vi "Helper - detect wind cross.vi"(10 "Heading Change":dbl, 11 "Apparent Wind":T1) -> (3 "Crossing Wind?":bool)   [LabVIEW 2011]
doc: "Checks whether the boat wants to cross the wind. Takes in the difference between optimal heading and current heading and the apparent wind. Returns true if the boat wants to cross the wind."
uses:
  2 Typedefs/apparent wind.ctl
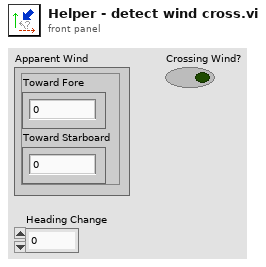
[diagram p1: front panel]
types:
  T1 = typedef "apparent wind.ctl" = cluster{"Toward Fore":dbl, "Toward Starboard":dbl}
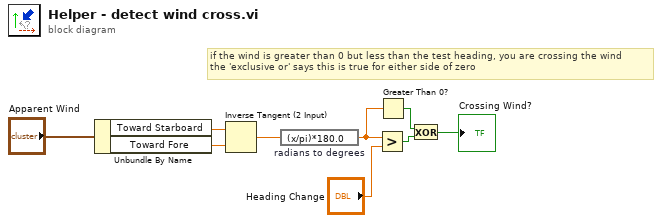
[diagram p0: block diagram]
diagram:
  # "if the wind is greater than 0 but less than the test heading, you are crossing the wind\nthe 'exclusive or' says this is true for either side of zero"
  n1 = Unbundle By Name("Apparent Wind") -> ("Toward Starboard"=w3:dbl, "Toward Fore"=w4:dbl)
  n2 = Inverse Tangent (2 Input)(1:w4, 2:w3) -> (0:w9:dbl)
  n3 = expression code="(x/pi)*180.0" "radians to degrees"(w9) -> (w6:dbl)
  n4 = Greater?(x=w6, y="Heading Change") -> (0:w7:bool)
  n5 = Greater Than 0?(x=w6) -> (x > 0?=w8:bool)
  n6 = Exclusive Or(1:w7, 2:w8) -> (0:→"Crossing Wind?":bool)
